vi "third version.vi"() -> ()   [LabVIEW 2015]
uses:
  <vilib>/Utility/NIReport.llb/Append Report Text (str wrap).vi
  <vilib>/Utility/NIReport.llb/NI_report.lvclass
panel:
  in  "SCAN HERE 2":string caption="Scan now"
  out "String":string
  in  "OK Button":bool
  in  "SCAN HERE":string caption="Scan now"
  in  "Cancel":bool
  out "STATUS":string
  out "MAC ID":string
  out "SERIAL NUMBER":string
  out "Program name":string
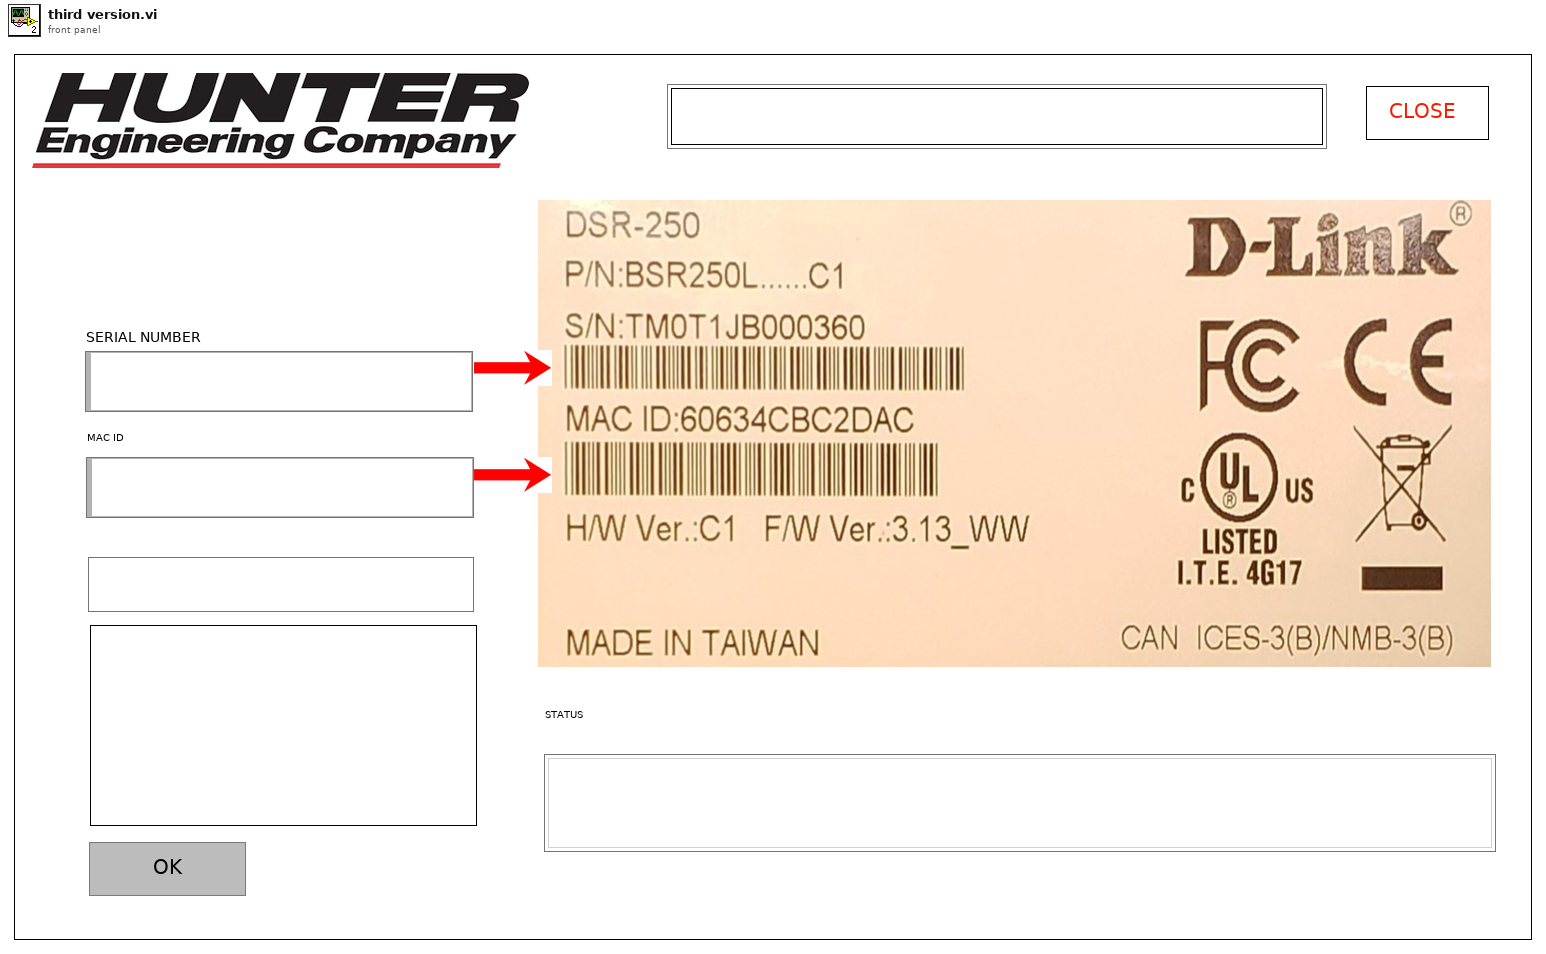
[diagram p1: front panel]
types:
  T1 = enum16{"Standard Report", "HTML", "Word", "Excel"}
  T2 = cluster{"Charset (-1)":i16, "Weight (-1)":i16, "Name":string, "Size":string}
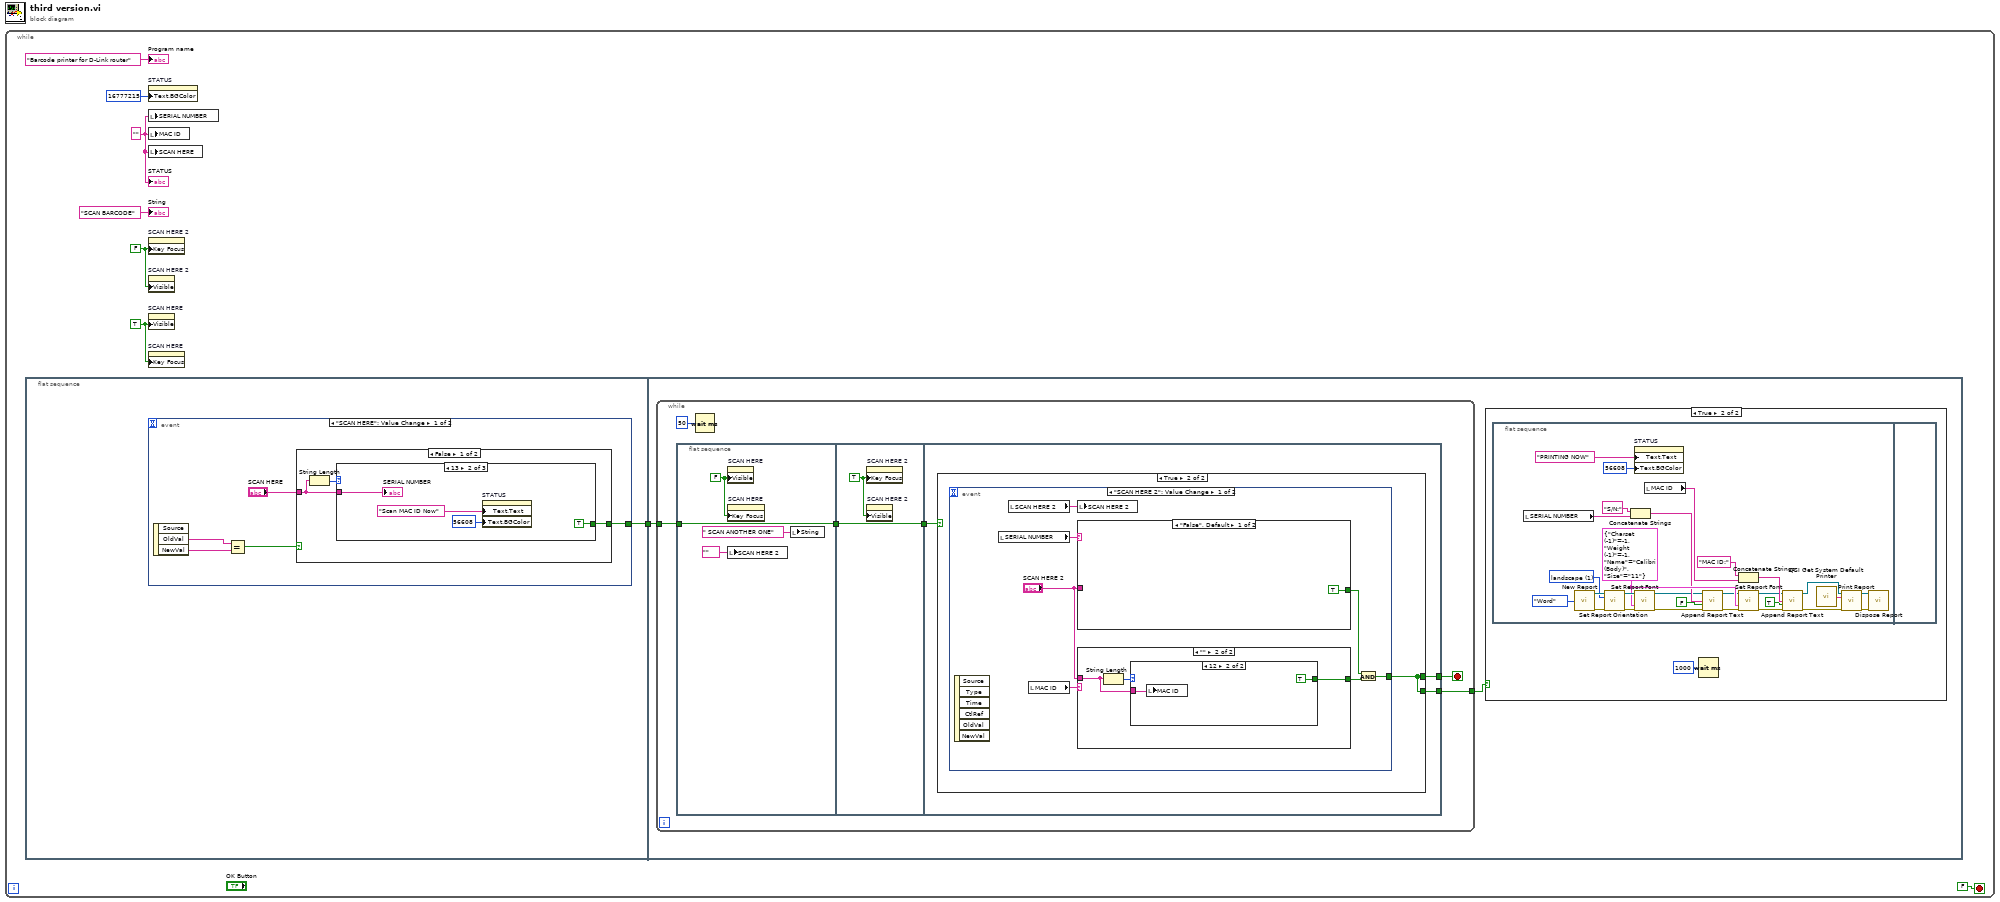
[diagram p0: block diagram]
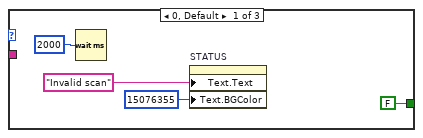
[diagram p2: hidden frame]
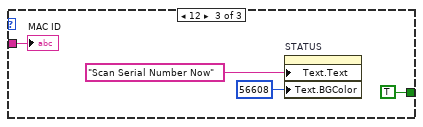
[diagram p3: hidden frame]
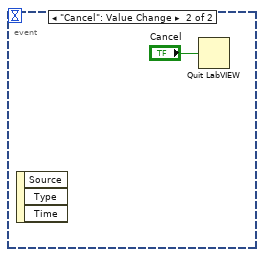
[diagram p5: hidden frame]
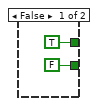
[diagram p7: hidden frame]
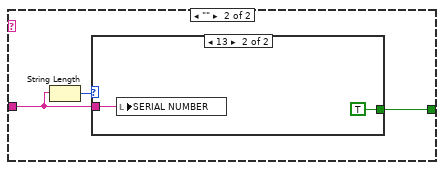
[diagram p8: hidden frame]
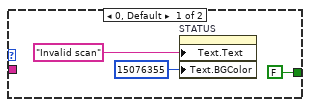
[diagram p9: hidden frame]
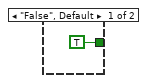
[diagram p10: hidden frame]
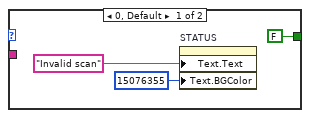
[diagram p11: hidden frame]
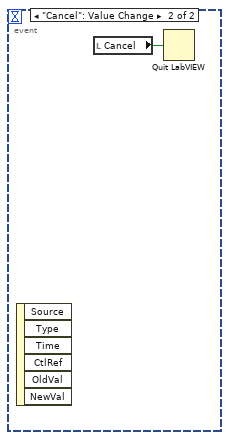
[diagram p12: hidden frame]
diagram:
  n1 = while {
    stop <- FALSE stop-if-true
    w3 = "" ("Serial Number")
    w6 = FALSE ("Key Focus")
    w5 = TRUE ("Visible")
    n2 = flat-sequence {
      tunnel: [w9] -> w7
      tunnel: w7 -> [w32]
      frame #0 {
        n3 = event shown="[0] \"SCAN HERE\": Value Change" {
          selector: _ -> [_ _]
          dyn-events: _ -> [_ _]
          timeout: _ -> [_ _]
          tunnel: [w11 _] -> w9
          event "SCAN HERE": Value Change {
            n4 = event-data() -> ("OldVal"=w14:string, "NewVal"=w13:string)  [unwired: 1 in, 1 out]
            n5 = Equal?(x=w14, y=w13) -> (x = y?=w12:bool)
            n6 = case shown="False" w12 {
              tunnel: "SCAN HERE" -> [w16 _]
              tunnel: [w15 _] -> w11
              frame False {
                n7 = String Length(string=w16) -> (length=w17:i32)
                n8 = case shown="13" w17 {
                  tunnel: w16 -> [_ w25 w29]
                  tunnel: [FALSE TRUE TRUE] -> w15
                  frame 0, Default {
                    n9 = Wait (ms)(milliseconds to wait=u32 2000) -> ()  [unwired: 1 out]
                    n10 = property on="STATUS" class="Str"("Text.Text"="Invalid scan", "Text.BGColor"=u32 15076355 ("Text.Text Colors:BG Color")) -> ()  [unwired: 2 in, 2 out]
                  }
                  frame 13 {
                    n11 = property on="STATUS" class="Str"("Text.Text"="Scan MAC ID Now" ("STATUS"), "Text.BGColor"=u32 56608 ("Text.Text Colors:BG Color")) -> ()  [unwired: 2 in, 2 out]
                    "SERIAL NUMBER" <- w25
                  }
                  frame 12 {
                    n12 = property on="STATUS" class="Str"("Text.Text"="Scan Serial Number Now" ("STATUS"), "Text.BGColor"=u32 56608 ("Text.Text Colors:BG Color")) -> ()  [unwired: 2 in, 2 out]
                    "MAC ID" <- w29
                  }
                }
              }
              frame True {
              }
            }
          }
          event "Cancel": Value Change {
            n13 = event-data() -> ()  [unwired: 1 in, 3 out]
            n14 = Quit LabVIEW(quit? (T)="Cancel") -> ()
          }
        }
      }
      frame #1 {
        n15 = while {
          tunnel: w32 -> [w62]
          tunnel: [w66] -> w31
          stop <- w65 stop-if-true
          n16 = flat-sequence {
            tunnel: [w68] -> w63
            tunnel: w62 -> [w68]
            tunnel: [w72] -> w64
            tunnel: w63 -> [w72]
            tunnel: [w76] -> w66
            tunnel: [w75] -> w65
            tunnel: w64 -> [w74]
            frame #0 {
              w71 = FALSE ("Visible")
              n17 = property on="SCAN HERE" class="Str"("Visible"=w71) -> ()  [unwired: 2 in, 2 out]
              n18 = property on="SCAN HERE" class="Str"("Key Focus"=w71) -> ()  [unwired: 2 in, 2 out]
              n19 = local write "SCAN HERE 2"("" ("Scan here 2")) -> ()
              n20 = local write "String"(" SCAN ANOTHER ONE" ("String")) -> ()
            }
            frame #1 {
              w73 = TRUE ("Key Focus")
              n21 = property on="SCAN HERE 2" class="Str"("Key Focus"=w73) -> ()  [unwired: 2 in, 2 out]
              n22 = property on="SCAN HERE 2" class="Str"("Visible"=w73) -> ()  [unwired: 2 in, 2 out]
            }
            frame #2 {
              n23 = case shown="True" w74 {
                tunnel: [FALSE w79] -> w76
                tunnel: [TRUE w79] -> w75
                frame False {
                }
                frame True {
                  n24 = event shown="[0] \"SCAN HERE 2\": Value Change" {
                    selector: _ -> [_ _]
                    dyn-events: _ -> [_ _]
                    timeout: _ -> [_ _]
                    tunnel: [w82 _] -> w79
                    event "SCAN HERE 2": Value Change {
                      n25 = event-data() -> ()  [unwired: 1 in, 6 out]
                      n26 = local read "SERIAL NUMBER"() -> (w86:string)
                      n27 = local read "SCAN HERE 2"() -> (w81:string)
                      n28 = local read "MAC ID"() -> (w84:string)
                      n29 = local write "SCAN HERE 2"(w81) -> ()
                      n30 = case shown="\"False\", Default" w86 {
                        tunnel: [TRUE w90] -> w85
                        tunnel: "SCAN HERE 2" -> [_ w88]
                        frame "False", Default {
                        }
                        frame "" {
                          n31 = String Length(string=w88) -> (length=w89:i32)
                          n32 = case shown="13" w89 {
                            tunnel: [FALSE TRUE] -> w90
                            tunnel: w88 -> [_ w94]
                            frame 0, Default {
                              n33 = property on="STATUS" class="Str"("Text.Text"="Invalid scan", "Text.BGColor"=u32 15076355 ("Text.Text Colors:BG Color")) -> ()  [unwired: 2 in, 2 out]
                            }
                            frame 13 {
                              n34 = local write "SERIAL NUMBER"(w94) -> ()
                            }
                          }
                        }
                      }
                      n35 = case shown="\"\"" w84 {
                        tunnel: [TRUE w99] -> w83
                        tunnel: "SCAN HERE 2" -> [_ w97]
                        frame "False", Default {
                        }
                        frame "" {
                          n36 = String Length(string=w97) -> (length=w98:i32)
                          n37 = case shown="12" w98 {
                            tunnel: [FALSE TRUE] -> w99
                            tunnel: w97 -> [_ w103]
                            frame 0, Default {
                              n38 = property on="STATUS" class="Str"("Text.Text"="Invalid scan", "Text.BGColor"=u32 15076355 ("Text.Text Colors:BG Color")) -> ()  [unwired: 2 in, 2 out]
                            }
                            frame 12 {
                              n39 = local write "MAC ID"(w103) -> ()
                            }
                          }
                        }
                      }
                      n40 = And(x=w85, y=w83) -> (x .and. y?=w82:bool)
                    }
                    event "Cancel": Value Change {
                      n41 = event-data() -> ()  [unwired: 1 in, 6 out]
                      n42 = local read "Cancel"() -> (w105:bool)
                      n43 = Quit LabVIEW(quit? (T)=w105) -> ()
                    }
                  }
                }
              }
            }
          }
          n44 = Wait (ms)(milliseconds to wait=u32 50) -> ()  [unwired: 1 out]
        }
        n45 = case shown="True" w31 {
          frame False {
          }
          frame True {
            n46 = flat-sequence {
              frame #0 {
                w57 = 1 items=["portrait", "landscape"] ("orientation (portrait)")
                w52 = T2 {"Charset (-1)"=-1, "Weight (-1)"=-1, "Name"="Calibri (Body)", "Size"="11"} ("font settings")
                n47 = local read "SERIAL NUMBER"() -> (w51:string)
                n48 = call <vilib>:"New Report.vi"("report type"=T1."Word") -> ("report out"=w60:refnum<class "NI_report.lvclass">, "error out"=w61:errorcluster)  [unwired: 13 in]
                n49 = call-dynamic "Set Report Orientation.vi"("report in"=w60, "orientation (portrait)"=w57, "error in (no error)"=w61) -> ("report out"=w58:refnum<class "NI_report.lvclass">, "error out"=w59:errorcluster)  [unwired: 11 in]
                n50 = Concatenate Strings("S/N:" ("string"), w51) -> (w45:string)
                n51 = property on="STATUS" class="Str"("Text.Text"="PRINTING NOW" ("STATUS"), "Text.BGColor"=u32 56608 ("Text.Text Colors:BG Color")) -> ()  [unwired: 2 in, 2 out]
                n52 = call-dynamic "Set Report Font.vi"("report in"=w58, "font settings"=w52, "error in (no error)"=w59) -> ("report out"=w41:refnum<class "NI_report.lvclass">, "error out"=w42:errorcluster)  [unwired: 10 in, 1 out]
                n53 = local read "MAC ID"() -> (w54:string)
                n54 = call-poly <vilib>:"Append Report Text.vi"("report in"=w41, "text"=w45, "append on new line? (F)"=FALSE, "error in (no error)"=w42) -> ("report out"=w38:refnum<class "NI_report.lvclass">, "error out"=w37:errorcluster)  [unwired: 8 in, 2 out]
                n55 = Concatenate Strings("MAC ID:" ("string"), w54) -> (w53:string)
                n56 = call-dynamic "Set Report Font.vi"("report in"=w38, "font settings"=w52, "error in (no error)"=w37) -> ("report out"=w50:refnum<class "NI_report.lvclass">, "error out"=w48:errorcluster)  [unwired: 10 in, 1 out]
                n57 = call-poly <vilib>:"Append Report Text.vi"("report in"=w50, "text"=w53, "append on new line? (F)"=TRUE, "error in (no error)"=w48) -> ("report out"=w36:refnum<class "NI_report.lvclass">, "error out"=w35:errorcluster)  [unwired: 8 in, 2 out]
                n58 = call "QSI Get System Default Printer.vi"() -> ("System Default Printer"=w34:string)  [unwired: 4 in, 1 out]
                n59 = call-dynamic "Print Report.vi"("report in"=w36, "printer name (default)"=w34, "error in (no error)"=w35) -> ("report out"=w40:refnum<class "NI_report.lvclass">, "error out"=w39:errorcluster)  [unwired: 11 in]
                n60 = call-dynamic "Dispose Report.vi"("report in"=w40, "error in (no error)"=w39) -> ()  [unwired: 13 in, 1 out]
              }
              frame #1 {
              }
            }
            n61 = Wait (ms)(milliseconds to wait=u32 1000) -> ()  [unwired: 1 out]
          }
        }
      }
    }
    n62 = property on="STATUS" class="Str"("Text.BGColor"=u32 16777215 ("Text.Text Colors:BG Color")) -> ()  [unwired: 2 in, 2 out]
    n63 = local write "SERIAL NUMBER"(w3) -> ()
    n64 = local write "MAC ID"(w3) -> ()
    n65 = local write "SCAN HERE"(w3) -> ()
    n66 = property on="SCAN HERE 2" class="Str"("Key Focus"=w6) -> ()  [unwired: 2 in, 2 out]
    n67 = property on="SCAN HERE 2" class="Str"("Visible"=w6) -> ()  [unwired: 2 in, 2 out]
    n68 = property on="SCAN HERE" class="Str"("Visible"=w5) -> ()  [unwired: 2 in, 2 out]
    n69 = property on="SCAN HERE" class="Str"("Key Focus"=w5) -> ()  [unwired: 2 in, 2 out]
    "STATUS" <- w3
    "Program name" <- "Barcode printer for D-Link router" ("Program name")
    "String" <- "SCAN BARCODE" ("String")
  }
